vi "Last Aperture Time Setter.vi"(0 "Aperture Time (s)":dbl, 11 "error in (no error)":errorcluster) -> (15 "error out":errorcluster)   [LabVIEW 2023, in "NI-568x RF Power Meter.lvlib" / "SG 2250 Path Accessor.lvclass"]
uses:
  SG 2250 Path Accessor.lvclass
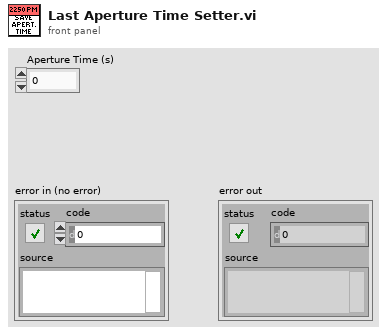
[diagram p1: front panel]
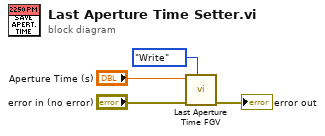
[diagram p0: block diagram]
diagram:
  n1 = call "Last Aperture Time FGV.vi"("Action"=enum16{"Write", "Read"}."Write", "error in (no error)"="error in (no error)", "Write Value (s)"="Aperture Time (s)") -> ("error out"=→"error out":errorcluster)  [unwired: 4 in, 1 out]
